vi "vroom calculator.vi"(11 "motor input":dbl) -> (2 "level of vroom":string, 3 "motor output":dbl)   [LabVIEW 2014]
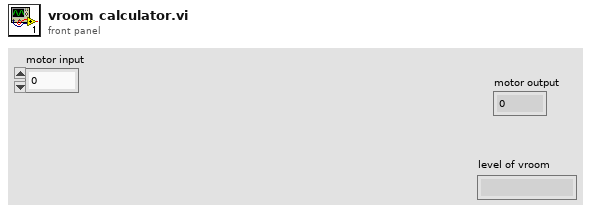
[diagram p1: front panel]
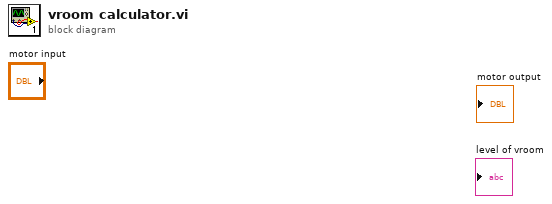
[diagram p0: block diagram]
diagram:
